vi "温度判别.vi"() -> ()   [LabVIEW 2018]
panel:
  out "s? t:f":string
  out "温度计":dbl(slide) scale=0.0..10.0
  in  "设置值":i32
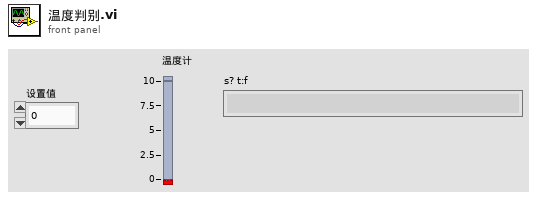
[diagram p1: front panel]
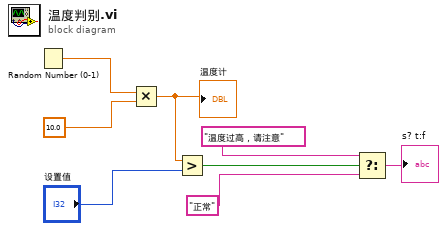
[diagram p0: block diagram]
diagram:
  n1 = Random Number (0-1)() -> (number: 0 to 1=w7:dbl)
  n2 = Multiply(x=w7, y=10.0) -> (x*y=w6:dbl)
  "温度计" <- w6
  n3 = Greater?(x=w6, y="设置值") -> (0:w4:bool)
  n4 = Select(t="温度过高，请注意", s=w4, f="正常") -> (s? t:f=→"s? t:f":string)
